vi "Traps-01-17.vi"(0 "Periode(us)":u32, 1 "zwischenMesswerten(us)":u16, 2 "Warten(us)":u16, 5 "5Van(us)":u16, 7 "HeizenTrap1":bool, 9 "Messwerte":i32, 11 "SPTrap1":fxp<+/-,16,6> format="%.12g", 12 "PIDTrap1":T1={"proportional gain (Kc)"=1.0, "integral gain (Kc*Ts/Ti)"=1.66796875, "derivative gain (Kc*Td/Ts)"=0.0} {"proportional gain (Kc)" format="%.11g"; "integral gain (Kc*Ts/Ti)" format="%.11g"; "derivative gain (Kc*Td/Ts)" format="%.11g"}) -> (4 "MWTrap1":fxp<+/-,27,6> format="%.23g", 8 "MWTrap2":fxp<+/-,27,6> format="%.23g")   [LabVIEW 2010]
uses:
  <vilib>/addons/control/pid/fpga.llb/XNode/niFpgaPID.xnode
  <vilib>/rvi/eio/common/nirviEmuClasses.ctl
  <vilib>/rvi/eio/common/nirviEmuTemplateMethod_noerrors.vi
  <vilib>/rvi/eio/nirviEIOImplementation/nirviEIOImplementation.xnode
  <vilib>/eio/EIONode/EIONode.xnode
  <vilib>/rvi/FXPMathLib/FxpDiv/XNode/nifxpmath_Div.xnode
  <vilib>/rvi/FXPMathLib/FxpAdd/XNode/nifxpmath_Add.xnode
  <vilib>/rvi/FXPMathLib/FxpDiv/simVIs/DllFxpDivTemp_sub.vi
  <vilib>/rvi/FXPMathLib/FxpDiv/subVIs/nifxpmath_Div_SimConfig.ctl
  <vilib>/fxp/LVFixedPointOverflowPolicyTypeDef.ctl
  <vilib>/fxp/LVFixedPointQuantizationPolicyTypeDef.ctl
  <vilib>/rvi/FXPMathLib/FxpConvert/XNode/nifxpmath_Convert.xnode
  <vilib>/rvi/FXPMathLib/FxpConvert/simVIs/DllFxpConvertTemp_sub.vi
  <vilib>/rvi/FXPMathLib/FxpConvert/subVIs/nifxpmath_Convert_SimConfig.ctl
  <vilib>/rvi/FXPMathLib/FxpMul/XNode/nifxpmath_Multiplier.xnode
  <vilib>/rvi/FXPMathLib/FxpMul/simVIs/DllFxpMulTemp_sub.vi
  <vilib>/rvi/FXPMathLib/FxpMul/subVIs/nifxpmath_Mul_SimConfig.ctl
  <vilib>/rvi/FXPMathLib/FxpAdd/simVIs/DllFxpAddTemp_sub.vi
  <vilib>/rvi/FXPMathLib/FxpAdd/subVIs/nifxpmath_Add_SimConfig.ctl
panel:
  in  "HeizenTrap2":bool
  in  "PIDTrap2":T1={"proportional gain (Kc)"=1.0, "integral gain (Kc*Ts/Ti)"=1.66796875, "derivative gain (Kc*Td/Ts)"=0.0} {"proportional gain (Kc)" format="%.11g"; "integral gain (Kc*Ts/Ti)" format="%.11g"; "derivative gain (Kc*Td/Ts)" format="%.11g"}
  in  "SPTrap2":fxp<+/-,16,6> format="%.12g"
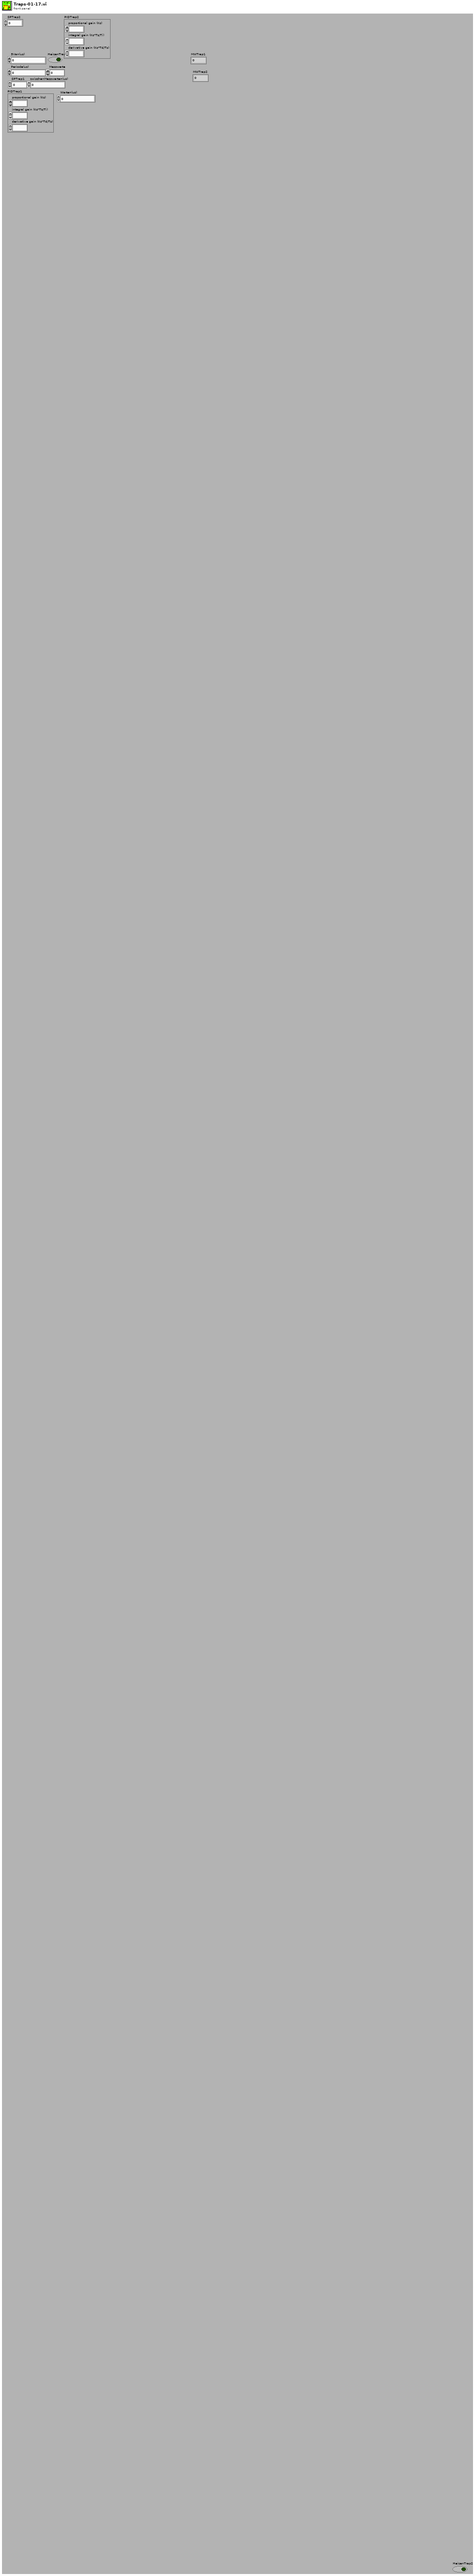
[diagram p1: front panel]
types:
  T1 = cluster{"proportional gain (Kc)":fxp<+/-,16,8>, "integral gain (Kc*Ts/Ti)":fxp<+/-,16,8>, "derivative gain (Kc*Td/Ts)":fxp<+/-,16,8>}
  T2 = typedef "nirviEmuClasses.ctl" = enum16{"IO Read", "IO Write", "Method", "Property Read", "Property Write"}
  T3 = cluster{"proportional gain (Kc)":i16, "integral gain (Kc*Ts/Ti)":i16, "derivative gain (Kc*Td/Ts)":i16}
  T4 = cluster{"output high":fxp<+/-,16,6>, "output low":fxp<+/-,16,6>}
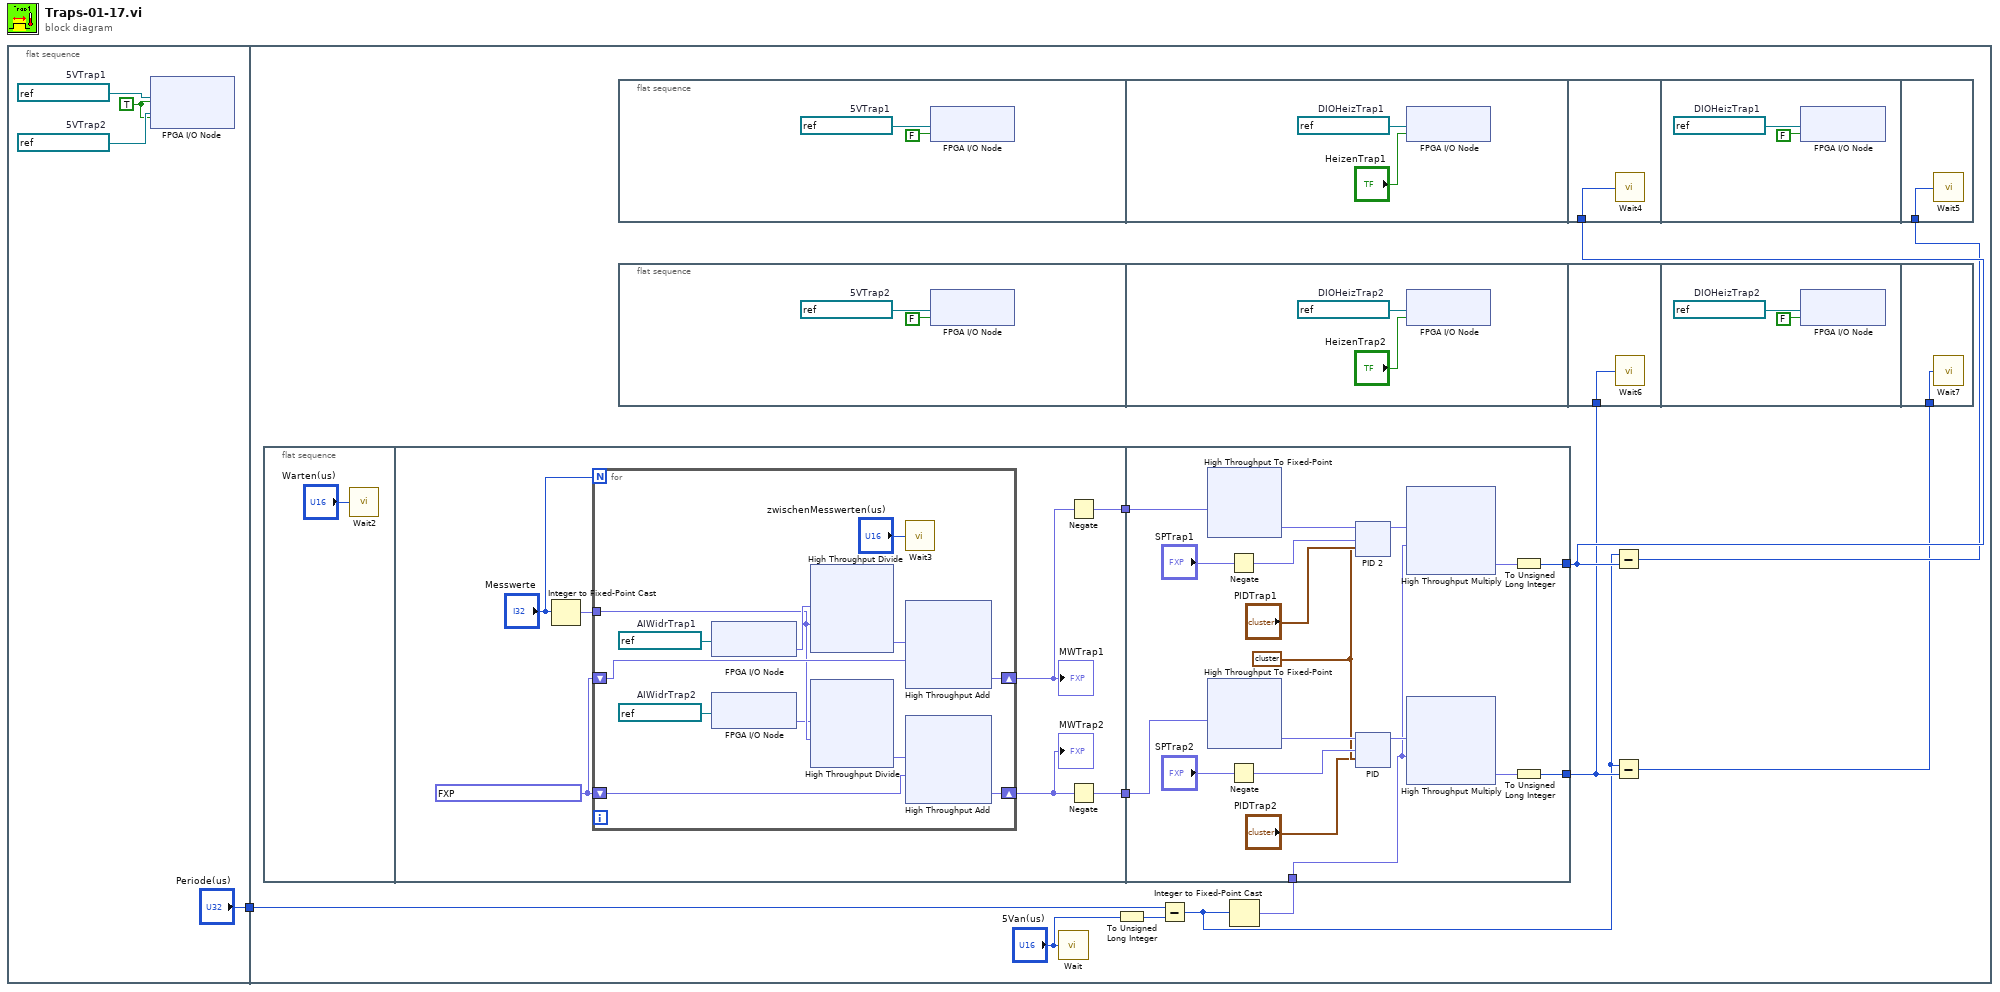
[diagram p0: block diagram]
diagram:
  n1 = flat-sequence {
    tunnel: ["Periode(us)"] -> w1
    tunnel: w1 -> [w10]
    frame #0 {
      w3 = refnum<k21> "Mod6/DIO21"  # 5VTrap2
      w2 = TRUE ("I/O Item")
      w4 = refnum<k21> "Mod6/DIO21"  # 5VTrap1
      n2 = xnode "FPGA I/O Node"("I/O Item"=w2, "I/O Item"=w2, "FPGA I/O In"=w4, "FPGA I/O In"=w3) -> ()  [unwired: 2 out]
    }
    frame #1 {
      n3 = flat-sequence {
        tunnel: [w22] -> w12
        tunnel: [w18] -> w11
        tunnel: w12 -> [w206]
        tunnel: w7 -> [w191]
        tunnel: [w201] -> w16
        tunnel: w11 -> [w199]
        tunnel: [w189] -> w14
        frame #0 {
          n4 = call "Wait2"("Count(uSec)"="Warten(us)") -> ()  [unwired: 1 out]
        }
        frame #1 {
          w20 = fxp<+/-,26,5> 0.0 ("I/O Item")
          n5 = Integer to Fixed-Point Cast(integer="Messwerte") -> (fixed-point=w23:fxp<+/-,32,32>)  [unwired: 1 in]
          n6 = for {
            N: "Messwerte" -> [_]
            shift-right: [w32] -> w21
            shift-left: w20 -> [w33]
            tunnel: w23 -> [w29]
            shift-right: [w25] -> w19
            shift-left: w20 -> [w26]
            w30 = refnum<k21> "Mod1/AI30"  # AIWidrTrap2
            w36 = refnum<k21> "Mod1/AI30"  # AIWidrTrap1
            n7 = xnode "FPGA I/O Node"("FPGA I/O In"=w36) -> ("I/O Item"=w35:fxp<+/-,26,5>)  [unwired: 1 out]
            n8 = xnode "FPGA I/O Node"("FPGA I/O In"=w30) -> ("I/O Item"=w28:fxp<+/-,26,5>)  [unwired: 1 out]
            n9 = xnode "High Throughput Divide"("x"=w35, "y"=w29) -> ("x/y"=w34:fxp<+/-,26,5>)
            n10 = xnode "High Throughput Divide"("x"=w28, "y"=w29) -> ("x/y"=w27:fxp<+/-,26,5>)
            n11 = call "Wait3"("Count(uSec)"="zwischenMesswerten(us)") -> ()  [unwired: 1 out]
            n12 = xnode "High Throughput Add"("x"=w34, "y"=w33) -> ("x+y"=w32:fxp<+/-,27,6>)
            n13 = xnode "High Throughput Add"("x"=w27, "y"=w26) -> ("x+y"=w25:fxp<+/-,27,6>)
          }
          "MWTrap1" <- w21
          "MWTrap2" <- w19
          n14 = Negate(x=w21) -> (-x=w22:fxp<+/-,28,7>)
          n15 = Negate(x=w19) -> (-x=w18:fxp<+/-,28,7>)
        }
        frame #2 {
          w194 = T4 {"output high"=1.0, "output low"=0.0} ("output range")
          n16 = xnode "High Throughput To Fixed-Point"("x"=w206) -> ("y"=w205:fxp<+/-,16,6>)
          n17 = xnode "High Throughput To Fixed-Point"("x"=w199) -> ("y"=w197:fxp<+/-,16,6>)
          n18 = Negate(x="SPTrap1") -> (-x=w196:fxp<+/-,16,6>)
          n19 = Negate(x="SPTrap2") -> (-x=w195:fxp<+/-,16,6>)
          n20 = xnode ("PID 2")("process variable"=w205, "setpoint"=w196, "PID gains"="PIDTrap1", "output range"=w194) -> ("output"=w203:fxp<+/-,16,6>)  [unwired: 1 in]
          n21 = xnode ("PID")("process variable"=w197, "setpoint"=w195, "PID gains"="PIDTrap2", "output range"=w194) -> ("output"=w192:fxp<+/-,16,6>)  [unwired: 1 in]
          n22 = xnode "High Throughput Multiply"("x"=w203, "y"=w191) -> ("x*y"=w202:fxp<+/-,32,32>)
          n23 = xnode "High Throughput Multiply"("x"=w192, "y"=w191) -> ("x*y"=w190:fxp<+/-,32,32>)
          n24 = To Unsigned Long Integer(number=w202) -> (unsigned 32bit integer=w201:u32)
          n25 = To Unsigned Long Integer(number=w190) -> (unsigned 32bit integer=w189:u32)
        }
      }
      n26 = flat-sequence {
        tunnel: w16 -> [w450]
        tunnel: w15 -> [w464]
        frame #0 {
          w425 = refnum<k21> "Mod6/DIO21"  # 5VTrap1
          n27 = xnode "FPGA I/O Node"("I/O Item"=FALSE, "FPGA I/O In"=w425) -> ()  [unwired: 1 out]
        }
        frame #1 {
          w437 = refnum<k21> "Mod6/DIO19"  # DIOHeizTrap1
          n28 = xnode "FPGA I/O Node"("I/O Item"="HeizenTrap1", "FPGA I/O In"=w437) -> ()  [unwired: 1 out]
        }
        frame #2 {
          n29 = call "Wait4"("Count(uSec)"=w450) -> ()  [unwired: 1 out]
        }
        frame #3 {
          w451 = refnum<k21> "Mod6/DIO19"  # DIOHeizTrap1
          n30 = xnode "FPGA I/O Node"("I/O Item"=FALSE, "FPGA I/O In"=w451) -> ()  [unwired: 1 out]
        }
        frame #4 {
          n31 = call "Wait5"("Count(uSec)"=w464) -> ()  [unwired: 1 out]
        }
      }
      n32 = flat-sequence {
        tunnel: w14 -> [w409]
        tunnel: w13 -> [w423]
        frame #0 {
          w384 = refnum<k21> "Mod6/DIO21"  # 5VTrap2
          n33 = xnode "FPGA I/O Node"("I/O Item"=FALSE, "FPGA I/O In"=w384) -> ()  [unwired: 1 out]
        }
        frame #1 {
          w396 = refnum<k21> "Mod6/DIO19"  # DIOHeizTrap2
          n34 = xnode "FPGA I/O Node"("I/O Item"="HeizenTrap2", "FPGA I/O In"=w396) -> ()  [unwired: 1 out]
        }
        frame #2 {
          n35 = call "Wait6"("Count(uSec)"=w409) -> ()  [unwired: 1 out]
        }
        frame #3 {
          w410 = refnum<k21> "Mod6/DIO19"  # DIOHeizTrap2
          n36 = xnode "FPGA I/O Node"("I/O Item"=FALSE, "FPGA I/O In"=w410) -> ()  [unwired: 1 out]
        }
        frame #4 {
          n37 = call "Wait7"("Count(uSec)"=w423) -> ()  [unwired: 1 out]
        }
      }
      n38 = call "Wait"("Count(uSec)"="5Van(us)") -> ()  [unwired: 1 out]
      n39 = To Unsigned Long Integer(number="5Van(us)") -> (unsigned 32bit integer=w8:u32)
      n40 = Subtract(x=w10, y=w8) -> (x-y=w6:u32)
      n41 = Integer to Fixed-Point Cast(integer=w6) -> (fixed-point=w7:fxp<+,32,32>)  [unwired: 1 in]
      n42 = Subtract(x=w6, y=w16) -> (x-y=w15:u32)
      n43 = Subtract(x=w6, y=w14) -> (x-y=w13:u32)
    }
  }
